vi "sub_strain-sum.vi"(11 "waveform history":waveform(dbl)[][](array[waveform])) -> (3 "원소 출력":waveform(dbl) caption="원소")   [LabVIEW 2013]
uses:
  <vilib>/Waveform/WDTOps.llb/WDT Append Waveforms DBL.vi
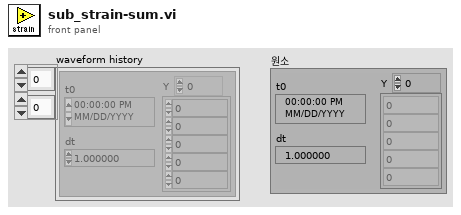
[diagram p1: front panel]
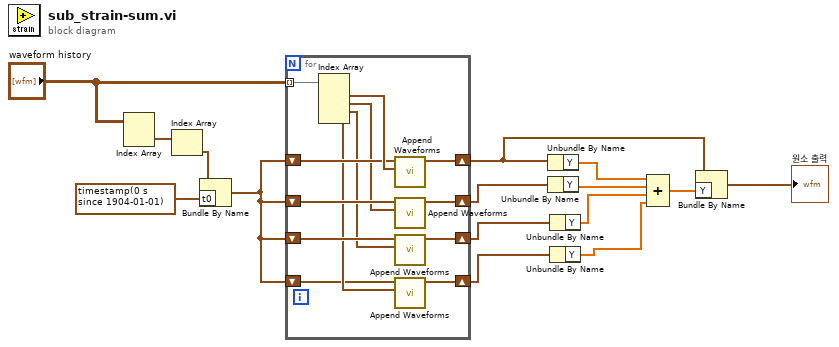
[diagram p0: block diagram]
diagram:
  n1 = Index Array(array="waveform history") -> (element=w4:waveform(dbl)[])  [unwired: 2 in]
  n2 = Index Array(array=w4) -> (element=w3:waveform(dbl))  [unwired: 1 in]
  n3 = Bundle By Name(cluster=w3, "t0"=timestamp(0 s since 1904-01-01)) -> (w1:waveform(dbl))
  n4 = for {
    tunnel: "waveform history" -> [w16] mode=indexing
    shift-right: [w28] -> w14
    shift-left: w1 -> [w23]
    shift-right: [w27] -> w11
    shift-left: w1 -> [w22]
    shift-right: [w26] -> w12
    shift-left: w1 -> [w20]
    shift-right: [w25] -> w13
    shift-left: w1 -> [w17]
    n5 = Index Array(array=w16) -> (element #1=w24:waveform(dbl), element #2=w21:waveform(dbl), element #3=w19:waveform(dbl), element #4=w18:waveform(dbl))  [unwired: 4 in]
    n6 = call-poly <vilib>:"Append Waveforms.vi"("waveform B"=w24, "waveform A"=w23) -> ("waveform out"=w28:waveform(dbl))  [unwired: 8 in, 1 out]
    n7 = call-poly <vilib>:"Append Waveforms.vi"("waveform B"=w21, "waveform A"=w22) -> ("waveform out"=w27:waveform(dbl))  [unwired: 8 in, 1 out]
    n8 = call-poly <vilib>:"Append Waveforms.vi"("waveform B"=w19, "waveform A"=w20) -> ("waveform out"=w26:waveform(dbl))  [unwired: 8 in, 1 out]
    n9 = call-poly <vilib>:"Append Waveforms.vi"("waveform B"=w18, "waveform A"=w17) -> ("waveform out"=w25:waveform(dbl))  [unwired: 8 in, 1 out]
  }
  n10 = Unbundle By Name(w14) -> ("Y"=w7:dbl[])
  n11 = Unbundle By Name(w11) -> ("Y"=w8:dbl[])
  n12 = Unbundle By Name(w12) -> ("Y"=w9:dbl[])
  n13 = Unbundle By Name(w13) -> ("Y"=w10:dbl[])
  n14 = Compound Arithmetic op=ADD(w7, w8, w9, w10) -> (w6:dbl[])
  n15 = Bundle By Name(cluster=w14, "Y"=w6) -> (→"원소 출력":waveform(dbl))
